vi "Clear errors mMc.vi"(1 "Port":T1={"P type"=0, "reference"="", " Terminator "="\r\n", "Timeout"=300} {"Timeout" step=10; "P type" items=["none", "RS-232C"]}, 3 "error in (no error)":errorcluster, 5 "Controller #":string) -> (9 "error out":errorcluster)   [LabVIEW 2011]
panel:
  # "Clear errors"
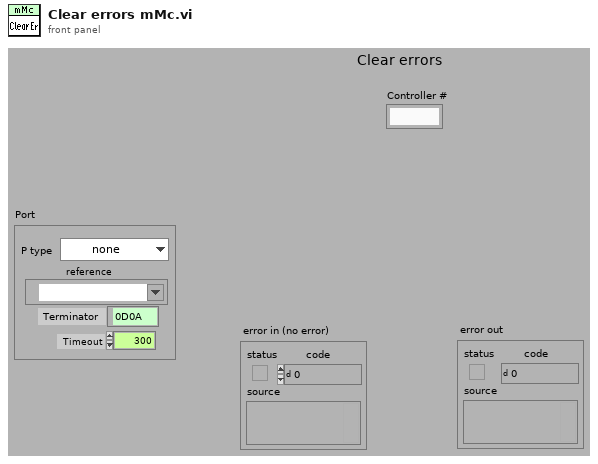
[diagram p1: front panel]
types:
  T1 = cluster{"P type":u16, "reference":refnum<visa-resource-name>, " Terminator ":string, "Timeout":i32}
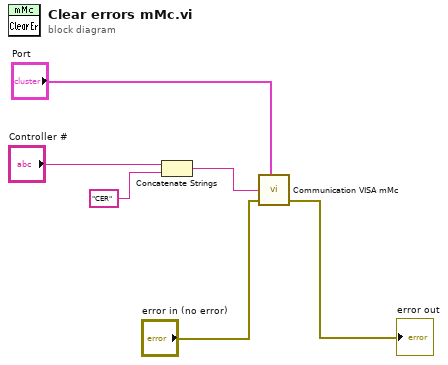
[diagram p0: block diagram]
diagram:
  n1 = Concatenate Strings("Controller #", "CER") -> (w2:string)
  n2 = call "Communication VISA mMc.vi"("Port"="Port", "Command"=w2, "error in (no error)"="error in (no error)") -> ("error out"=→"error out":errorcluster)  [unwired: 3 in, 3 out]
